vi "draw_to_matlab.vi"(4 "Z matrix":dbl[][](array[numeric]), 5 "draw to matlab":bool, 6 "y vector":dbl[](array[numeric]), 7 "plot to Matlab":bool, 9 "x vector":dbl[](array[numeric]), 10 "scatter to Matlab":bool, 11 "XYGraph in":refnum<vi>) -> ()   [LabVIEW 2015]
doc: "Copyright (c) 2018 Frans Korhonen, Institute for Atmospheric and Earth System Research / Physics, Faculty of Science, University of Helsinki, Finland\n\nThis file is part of MeasGUI.\n\nThis Source Code Form is subject to the terms of the Mozilla Public\nLicense, v. 2.0. If a copy of the MPL was not distributed with this\n file, You can obtain one at http://mozilla.org/MPL/2.0/."
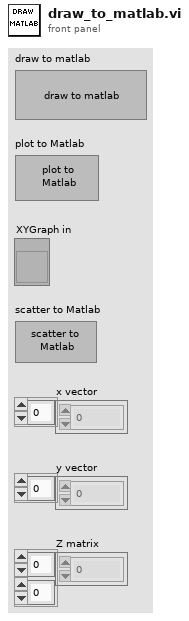
[diagram p1: front panel]
types:
  T1 = cluster{"measurement data":dbl[], "measurement data":dbl[]}[]
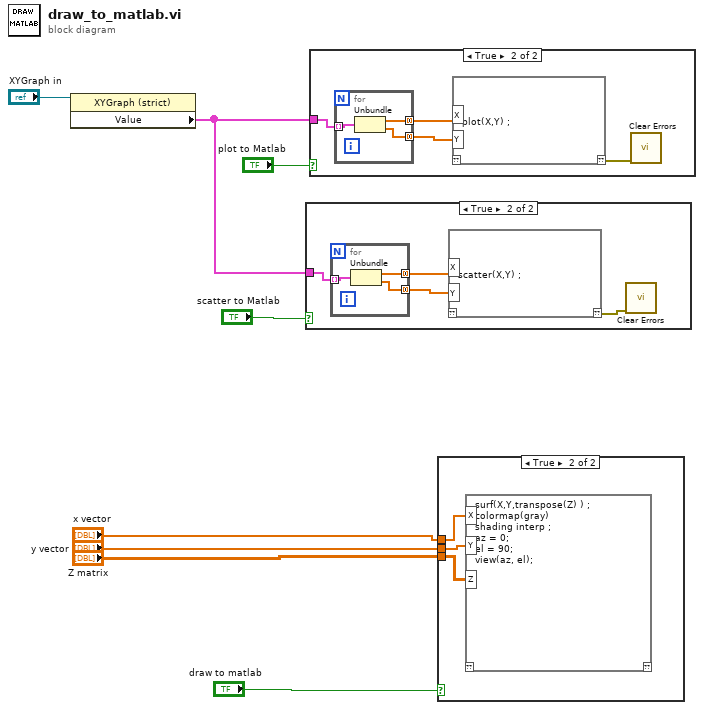
[diagram p0: block diagram]
diagram:
  n1 = property on="Property Node" class="XYGraph (strict)"(reference="XYGraph in") -> ("Value"=w5:T1)  [unwired: 1 in, 2 out]
  n2 = case shown="True" "scatter to Matlab" {
    tunnel: w5 -> [_ w9]
    frame False {
    }
    frame True {
      n3 = for {
        tunnel: w9 -> [w15] mode=indexing
        tunnel: [w14] -> w11 mode=concatenating
        tunnel: [w13] -> w10 mode=concatenating
        n4 = Unbundle(w15) -> ("measurement data"=w14:dbl[], "measurement data"=w13:dbl[])
      }
      n5 = script code="scatter(X,Y) ;"("X"=w11, "Y"=w10) -> ("??"=w12:errorcluster)  [unwired: 1 in]
      n6 = call <vilib>:"Clear Errors.vi"("error in (no error)"=w12) -> ()  [unwired: 5 in, 2 out]
    }
  }
  n7 = case shown="True" "plot to Matlab" {
    tunnel: w5 -> [_ w16]
    frame False {
    }
    frame True {
      n8 = for {
        tunnel: w16 -> [w22] mode=indexing
        tunnel: [w21] -> w18 mode=concatenating
        tunnel: [w20] -> w17 mode=concatenating
        n9 = Unbundle(w22) -> ("measurement data"=w21:dbl[], "measurement data"=w20:dbl[])
      }
      n10 = script code="plot(X,Y) ;"("X"=w18, "Y"=w17) -> ("??"=w19:errorcluster)  [unwired: 1 in]
      n11 = call <vilib>:"Clear Errors.vi"("error in (no error)"=w19) -> ()  [unwired: 5 in, 2 out]
    }
  }
  n12 = case shown="True" "draw to matlab" {
    tunnel: "x vector" -> [_ w25]
    tunnel: "Z matrix" -> [_ w23]
    tunnel: "y vector" -> [_ w24]
    frame False {
    }
    frame True {
      n13 = script code="surf(X,Y,transpose(Z) ) ;\ncolormap(gray)\nshading interp ;\naz = 0;\nel = 90;\nview(az, el);"("X"=w25, "Y"=w24, "Z"=w23) -> ()  [unwired: 1 in, 1 out]
    }
  }
